vi "Calculate TIFF page number.vi"(4 "Channel to process":enum16{"Red", "Green"}(ring), 8 "Global cycle index":i32, 9 "Number of planes":i32, 11 "Folder path":path) -> (1 "Page":u32, 3 "File path":path)   [LabVIEW 2017]
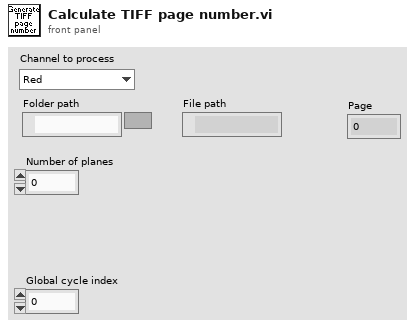
[diagram p1: front panel]
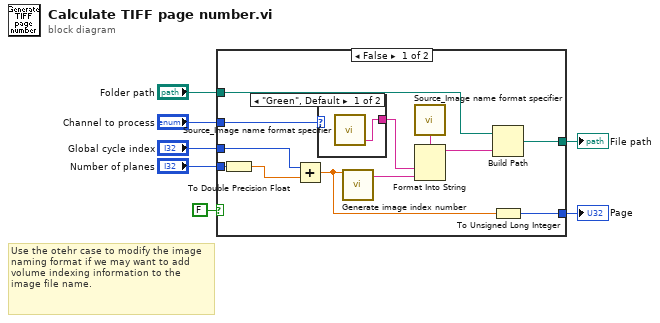
[diagram p0: block diagram]
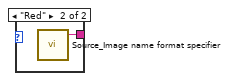
[diagram p2: hidden frame]
diagram:
  # "Use the otehr case to modify the image naming format if we may want to add volume indexing information to the image file name."
  n1 = case shown="False" FALSE {
    tunnel: "Global cycle index" -> [w19 _]
    tunnel: "Number of planes" -> [w18 _]
    tunnel: [w17 w22] -> w5
    tunnel: "Folder path" -> [w16 w22]
    tunnel: "Channel to process" -> [w11 _]
    tunnel: [w9 _] -> w1
    frame False {
      n2 = To Double Precision Float(number=w18) -> (double precision float=w8:dbl)
      n3 = Add(x=w19, y=w8) -> (x+y=w10:dbl)
      n4 = case shown="\"Green\", Default" w11 {
        tunnel: [w20 w21] -> w13
        frame "Green", Default {
          n5 = call "Source_Image name format specifier.vi"() -> ("Green channel name"=w20:string)  [unwired: 5 in, 2 out]
        }
        frame "Red" {
          n6 = call "Source_Image name format specifier.vi"() -> ("Red channel name"=w21:string)  [unwired: 5 in, 2 out]
        }
      }
      n7 = call "Generate image index number.vi"("FOR loop iteration or existing number of files"=w10) -> ("Number in string representation (padded with zeroes)"=w12:string)  [unwired: 10 in]
      n8 = call "Source_Image name format specifier.vi"() -> ("Z-Stack Image name format specifier"=w14:string)  [unwired: 5 in, 2 out]
      n9 = Format Into String(format string=w14, w13, w12) -> (resulting string=w15:string)  [unwired: 2 in, 1 out]
      n10 = Build Path(base path=w16, name or relative path=w15) -> (appended path=w17:path)
      n11 = To Unsigned Long Integer(number=w10) -> (unsigned 32bit integer=w9:u32)
    }
    frame True {
    }
  }
  "File path" <- w5
  "Page" <- w1
